vi "CRYPIC Replace FRAME.vi"(10 "tFrame":T2) -> (2 "tFrame_Out":T2)   [LabVIEW 2013]
uses:
  <vilib>/Utility/miscctls.llb/LVRectTypeDef.ctl
  CRYMain Sub Window Global.vi
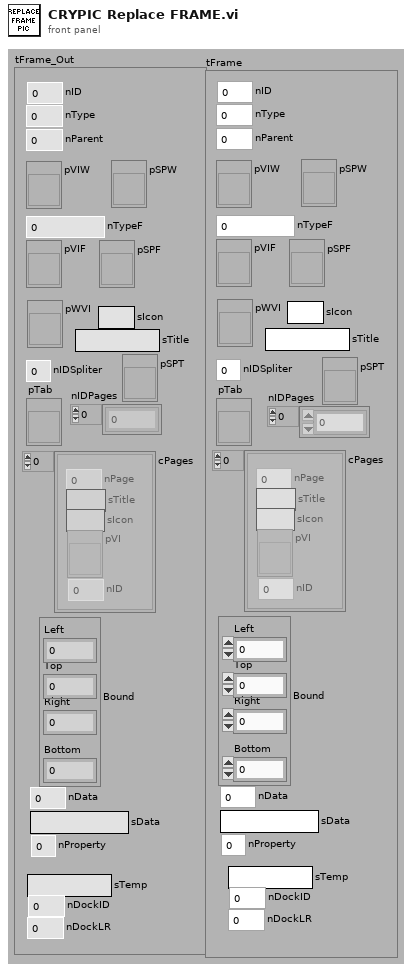
[diagram p1: front panel]
types:
  T1 = typedef "LVRectTypeDef.ctl" = cluster{"Left":i16, "Top":i16, "Right":i16, "Bottom":i16}
  T2 = cluster{"nType":i32, "nParent":i32, "pVIW":refnum<vi>, "pSPW":refnum<vi>, "nTypeF":i32, "pVIF":refnum<vi>, "pSPF":refnum<vi>, "nIDSpliter":i32, "nProperty":i32, "Bound":T1, "nID":i32, "nData":i32, "sData":string, "pWVI":refnum<vi>, "sTitle":string, "cPages":cluster{"nPage":i32, "sTitle":string, "sIcon":string, "pVI":refnum<vi>, "nID":i32}[], "pTab":refnum<vi>, "nIDPages":i32[], "pSPT":refnum<vi>, "sTemp":string, "nDockID":i32, "nDockLR":i32, "sIcon":string}
  T3 = cluster{"nID":i32[], "Frame":cluster{"nType":i32, "nParent":i32, "pVIW":refnum<vi>, "pSPW":refnum<vi>, "nTypeF":i32, "pVIF":refnum<vi>, "pSPF":refnum<vi>, "nIDSpliter":i32, "nProperty":i32, "Bound":T1, "nID":i32, "nData":i32, "sData":string, "pWVI":refnum<vi>, "sTitle":string, "cPages":cluster{"nPage":i32, "sTitle":string, "sIcon":string, "pVI":refnum<vi>, "nID":i32}[], "pTab":refnum<vi>, "nIDPages":i32[], "pSPT":refnum<vi>, "sTemp":string, "nDockID":i32, "nDockLR":i32, "sIcon":string}[]}
  T4 = cluster{"nType":i32, "nParent":i32, "pVIW":refnum<vi>, "pSPW":refnum<vi>, "nTypeF":i32, "pVIF":refnum<vi>, "pSPF":refnum<vi>, "nIDSpliter":i32, "nProperty":i32, "Bound":T1, "nID":i32, "nData":i32, "sData":string, "pWVI":refnum<vi>, "sTitle":string, "cPages":cluster{"nPage":i32, "sTitle":string, "sIcon":string, "pVI":refnum<vi>, "nID":i32}[], "pTab":refnum<vi>, "nIDPages":i32[], "pSPT":refnum<vi>, "sTemp":string, "nDockID":i32, "nDockLR":i32, "sIcon":string}[]
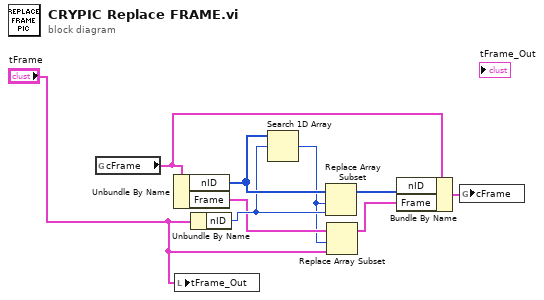
[diagram p0: block diagram]
diagram:
  n1 = global read "CRYMain Sub Window Global.vi" "cFrame"() -> (w7:T3)
  n2 = Unbundle By Name(w7) -> ("nID"=w6:i32[], "Frame"=w3:T4)
  n3 = local write "tFrame_Out"("tFrame") -> ()
  n4 = Unbundle By Name("tFrame") -> ("nID"=w5:i32)
  n5 = Search 1D Array(1D array=w6, element=w5) -> (index of element=w2:i32)  [unwired: 1 out]
  n6 = Replace Array Subset(array=w6, new element=w5, index=w2) -> (w8:i32[])
  n7 = Replace Array Subset(array=w3, new element="tFrame", index=w2) -> (w4:T4)
  n8 = Bundle By Name(cluster=w7, "nID"=w8, "Frame"=w4) -> (w9:T3)
  n9 = global write "CRYMain Sub Window Global.vi" "cFrame"(w9) -> ()
